vi "Cluster Typedef JSON Staging.vi"(8 "error in (no error)":errorcluster) -> (0 "error out":errorcluster, 1 "Experiment Description 2":T1, 2 "JSON String":string)   [LabVIEW 2016]
uses:
  <userlib>/LevyLab/Lockin-Multichannel/Typedefs/AO-cluster.ctl
  <userlib>/LevyLab/Lockin-Multichannel/Typedefs/AO_Amp-array.ctl
  <userlib>/LevyLab/Lockin-Multichannel/Typedefs/AO_DC-array.ctl
  <userlib>/LevyLab/Lockin-Multichannel/Typedefs/AO_f-array.ctl
  <userlib>/LevyLab/Lockin-Multichannel/Typedefs/AO_phi-array.ctl
  <userlib>/LevyLab/Lockin-Multichannel/Typedefs/Function-array.ctl
  <userlib>/LevyLab/Lockin-Multichannel/Typedefs/Function-enum.ctl
  <userlib>/LevyLab/Krohn Hite 7008/typedefs/KH_control_array.ctl
  <userlib>/LevyLab/Krohn Hite 7008/typedefs/KH_control.ctl
  <userlib>/LevyLab/Krohn Hite 7008/typedefs/Channel-Enum.ctl
  <userlib>/LevyLab/Krohn Hite 7008/typedefs/Gain-Enum.ctl
  <userlib>/LevyLab/Krohn Hite 7008/typedefs/Shunt-Enum.ctl
  <userlib>/LevyLab/Krohn Hite 7008/typedefs/Input Configuration-Enum.ctl
  <userlib>/LevyLab/Lockin-Multichannel/Typedefs/REF-cluster.ctl
  <userlib>/LevyLab/Lockin-Multichannel/Typedefs/REF_f-array.ctl
  <userlib>/LevyLab/Lockin-Multichannel/Typedefs/REF_phi-array.ctl
  <vilib>/addons/_JKI.lib/Serialization/JSON/JKI JSON Serialization.lvlib
  <userlib>/LevyLab/Krohn Hite 7008/KH7008.lvclass
  Control Experiment/Control Experiment.lvclass
panel:
  out "x = y?":T2
  out "from JSON (ms)":u32
  out "to JSON (ms)":u32
  in  "Experiment Description":T1
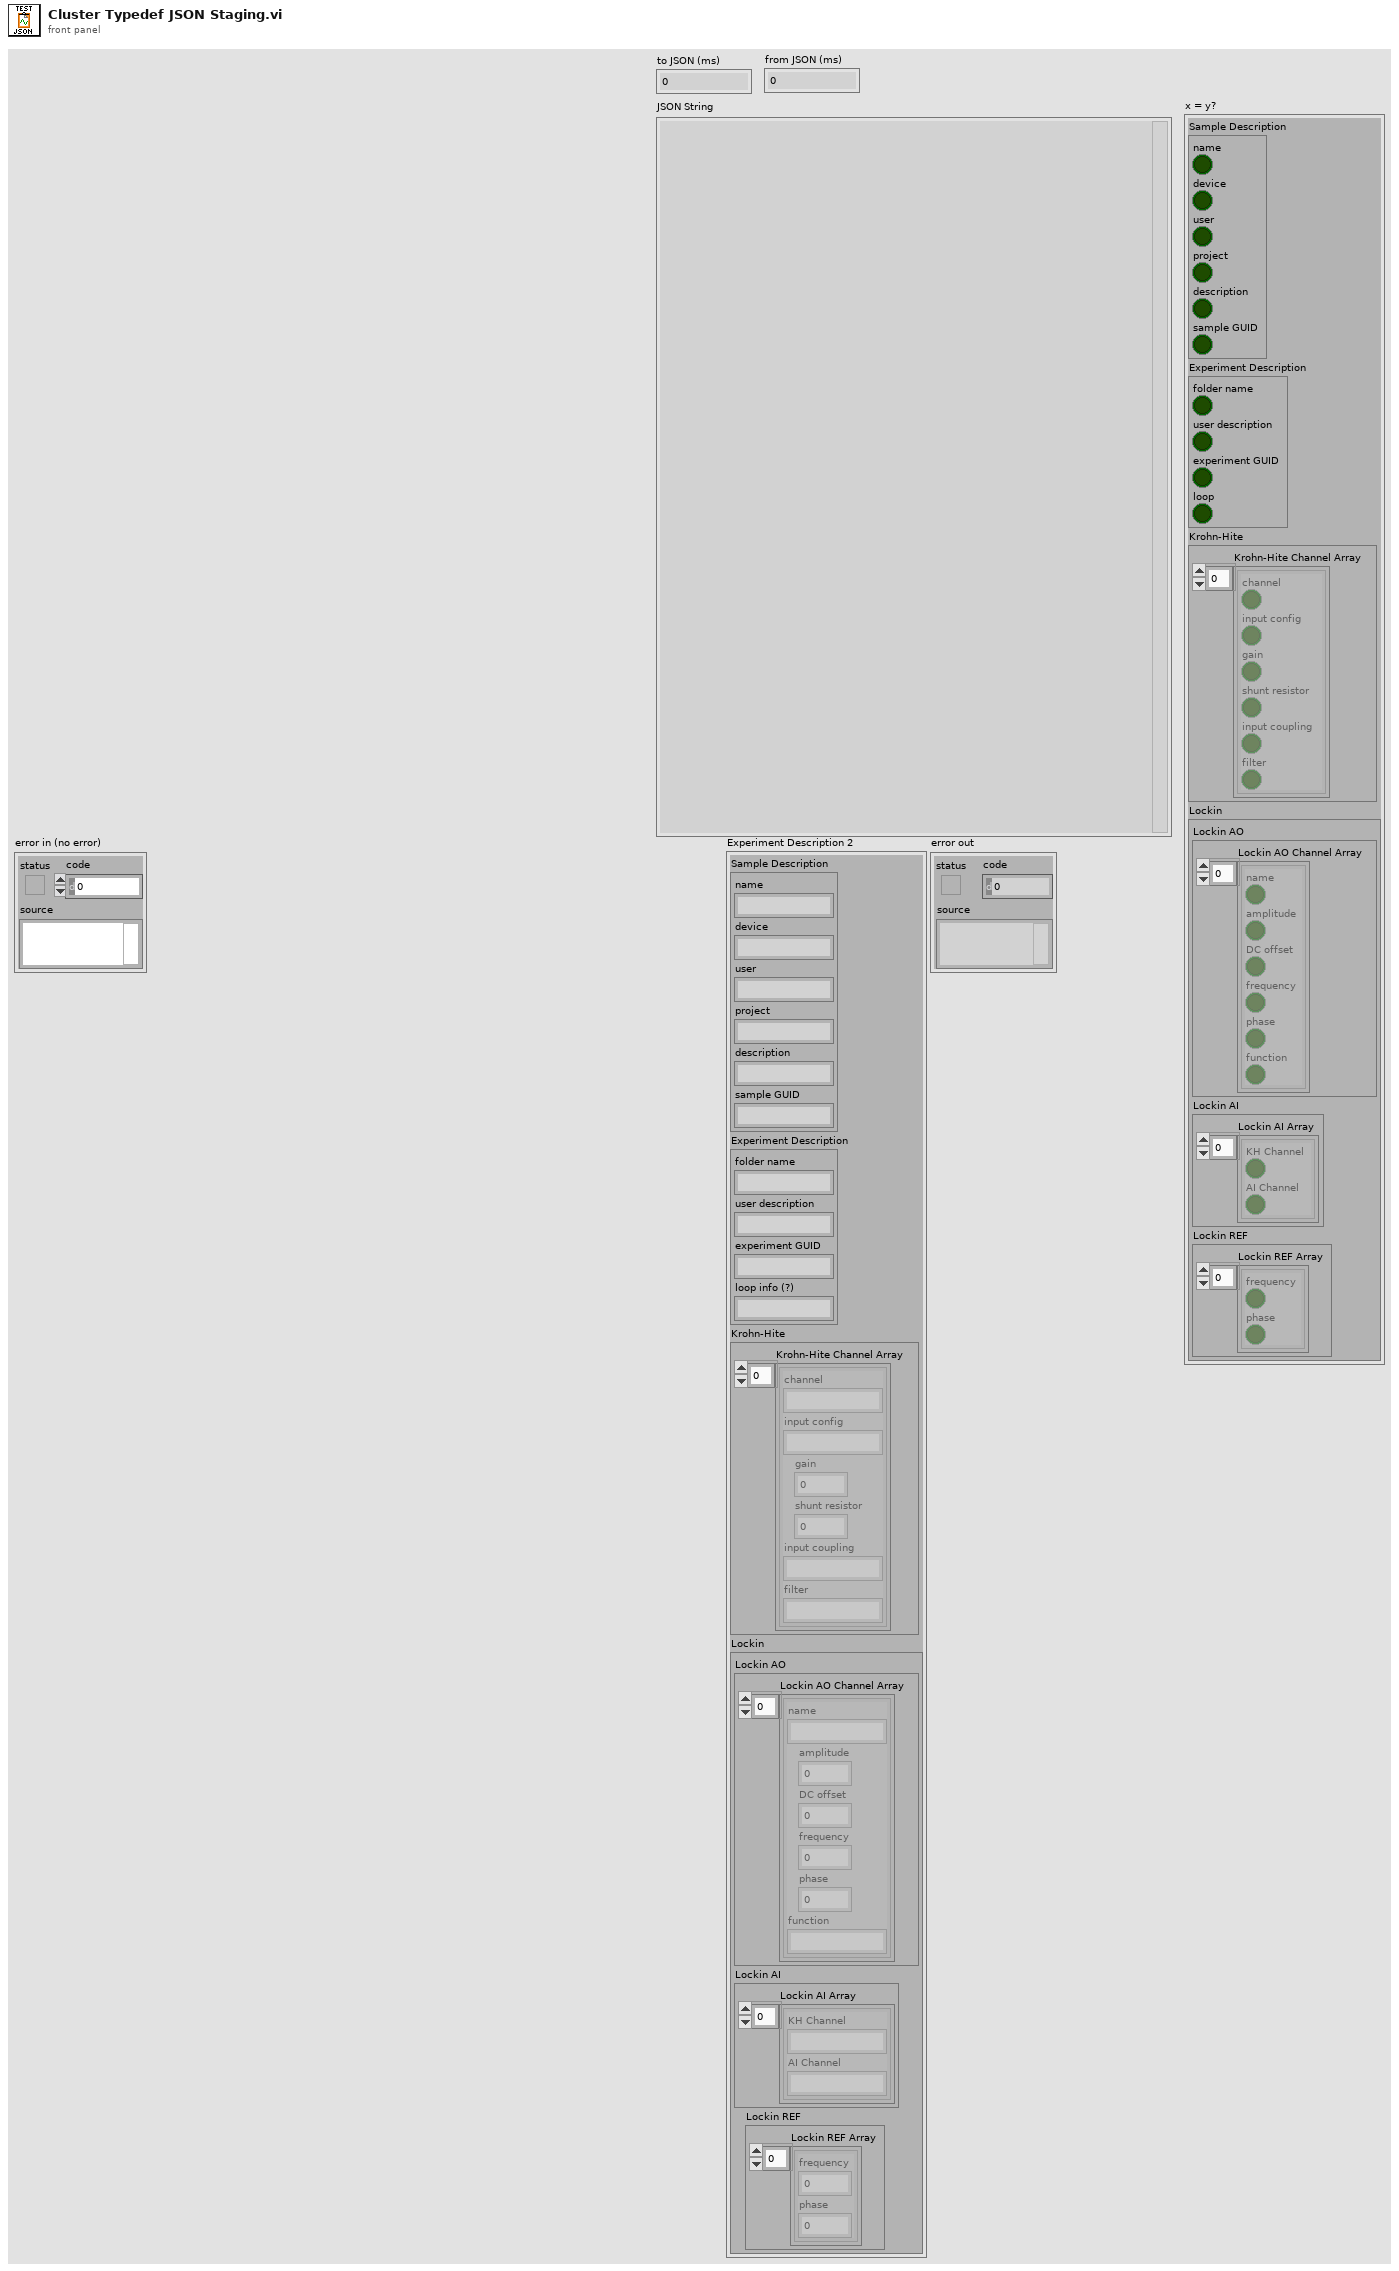
[diagram p1: front panel]
types:
  T1 = cluster{"Sample Description":cluster{"name":string, "device":string, "user":string, "project":string, "description":string, "sample GUID":string}, "Experiment Description":cluster{"folder name":string, "user description":string, "experiment GUID":string, "loop info (?)":string}, "Krohn-Hite":cluster{"Krohn-Hite Channel Array":cluster{"channel":string, "input config":string, "gain":i32, "shunt resistor":i32, "input coupling":string, "filter":string}[]}, "Lockin":cluster{"Lockin AO":cluster{"Lockin AO Channel Array":cluster{"name":string, "amplitude":dbl, "DC offset":dbl, "frequency":dbl, "phase":dbl, "function":string}[]}, "Lockin AI":cluster{"Lockin AI Array":cluster{"KH Channel":string, "AI Channel":string}[]}, "Lockin REF":cluster{"Lockin REF Array":cluster{"frequency":dbl, "phase":dbl}[]}}}
  T2 = cluster{"Sample Description":cluster{"name":bool, "device":bool, "user":bool, "project":bool, "description":bool, "sample GUID":bool}, "Experiment Description":cluster{"folder name":bool, "user description":bool, "experiment GUID":bool, "loop":bool}, "Krohn-Hite":cluster{"Krohn-Hite Channel Array":cluster{"channel":bool, "input config":bool, "gain":bool, "shunt resistor":bool, "input coupling":bool, "filter":bool}[]}, "Lockin":cluster{"Lockin AO":cluster{"Lockin AO Channel Array":cluster{"name":bool, "amplitude":bool, "DC offset":bool, "frequency":bool, "phase":bool, "function":bool}[]}, "Lockin AI":cluster{"Lockin AI Array":cluster{"KH Channel":bool, "AI Channel":bool}[]}, "Lockin REF":cluster{"Lockin REF Array":cluster{"frequency":bool, "phase":bool}[]}}}
  T3 = typedef "REF-cluster.ctl" = cluster{"REF f (Hz)":T4, "REF phi (°)":T5}
  T4 = typedef "REF_f-array.ctl" = dbl[]
  T5 = typedef "REF_phi-array.ctl" = dbl[]
  T6 = typedef "KH7008.lvclass/KH_control_array.ctl" = T7[]
  T7 = typedef "KH7008.lvclass/KH_control.ctl" = cluster{"Channel":T8, "Gain":T9, "Shunt Resistor":T10, "Input Config":T11}
  T8 = typedef "KH7008.lvclass/Channel-Enum.ctl" = enum16{"Channel 1", "Channel 2", "Channel 3", "Channel 4", "Channel 5", "Channel 6", "Channel 7", "Channel 8"}
  T9 = typedef "KH7008.lvclass/Gain-Enum.ctl" = enum16{"1x", "10x", "100x", "1000x"}
  T10 = typedef "KH7008.lvclass/Shunt-Enum.ctl" = enum16{"Open", "50 Ohms", "500 Ohms", "5k Ohms", "50k Ohms"}
  T11 = typedef "KH7008.lvclass/Input Configuration-Enum.ctl" = enum16{"Ground", "SE+ (-gnd)", "SE- (+gnd)", "Differential"}
  T12 = typedef "AO-cluster.ctl" = cluster{"AO amp (V)":T13, "AO DC (V)":T14, "AO f (Hz)":T15, "AO phi (°)":T16, "function":T17, "I+":bool[]}
  T13 = typedef "AO_Amp-array.ctl" = dbl[]
  T14 = typedef "AO_DC-array.ctl" = dbl[]
  T15 = typedef "AO_f-array.ctl" = dbl[]
  T16 = typedef "AO_phi-array.ctl" = dbl[]
  T17 = typedef "Function-array.ctl" = T18[]
  T18 = typedef "Function-enum.ctl" = enum16{"Sine", "Triangle", "Square", "Sawtooth"}
  T19 = cluster{"name":string, "device":string, "user":string, "project":string, "description":string, "sample GUID":string}
  T20 = cluster{"folder name":string, "user description":string, "experiment GUID":string, "loop info (?)":string}
  T21 = cluster{"Krohn-Hite Channel Array":cluster{"channel":string, "input config":string, "gain":i32, "shunt resistor":i32, "input coupling":string, "filter":string}[]}
  T22 = cluster{"Lockin AO":cluster{"Lockin AO Channel Array":cluster{"name":string, "amplitude":dbl, "DC offset":dbl, "frequency":dbl, "phase":dbl, "function":string}[]}, "Lockin AI":cluster{"Lockin AI Array":cluster{"KH Channel":string, "AI Channel":string}[]}, "Lockin REF":cluster{"Lockin REF Array":cluster{"frequency":dbl, "phase":dbl}[]}}
  T23 = cluster{"Lockin AO Channel Array":cluster{"name":string, "amplitude":dbl, "DC offset":dbl, "frequency":dbl, "phase":dbl, "function":string}[]}
  T24 = cluster{"Lockin REF Array":cluster{"frequency":dbl, "phase":dbl}[]}
  T25 = cluster{"Lockin AI Array":cluster{"KH Channel":string, "AI Channel":string}[]}
  T26 = cluster{"channel":string, "input config":string, "gain":i32, "shunt resistor":i32, "input coupling":string, "filter":string}[]
  T27 = cluster{"channel":string, "input config":string, "gain":i32, "shunt resistor":i32, "input coupling":string, "filter":string}
  T28 = cluster{"name":string, "amplitude":dbl, "DC offset":dbl, "frequency":dbl, "phase":dbl, "function":string}[]
  T29 = cluster{"name":string, "amplitude":dbl, "DC offset":dbl, "frequency":dbl, "phase":dbl, "function":string}
  T30 = cluster{"KH Channel":string, "AI Channel":string}[]
  T31 = cluster{"KH Channel":string, "AI Channel":string}
  T32 = cluster{"Sample Description":cluster{"name":bool, "device":bool, "user":bool, "project":bool, "description":bool, "sample GUID":bool}, "Experiment Description":cluster{"folder name":bool, "user description":bool, "experiment GUID":bool, "loop info (?)":bool}, "Krohn-Hite":cluster{"Krohn-Hite Channel Array":cluster{"channel":bool, "input config":bool, "gain":bool, "shunt resistor":bool, "input coupling":bool, "filter":bool}[]}, "Lockin":cluster{"Lockin AO":cluster{"Lockin AO Channel Array":cluster{"name":bool, "amplitude":bool, "DC offset":bool, "frequency":bool, "phase":bool, "function":bool}[]}, "Lockin AI":cluster{"Lockin AI Array":cluster{"KH Channel":bool, "AI Channel":bool}[]}, "Lockin REF":cluster{"Lockin REF Array":cluster{"frequency":bool, "phase":bool}[]}}}
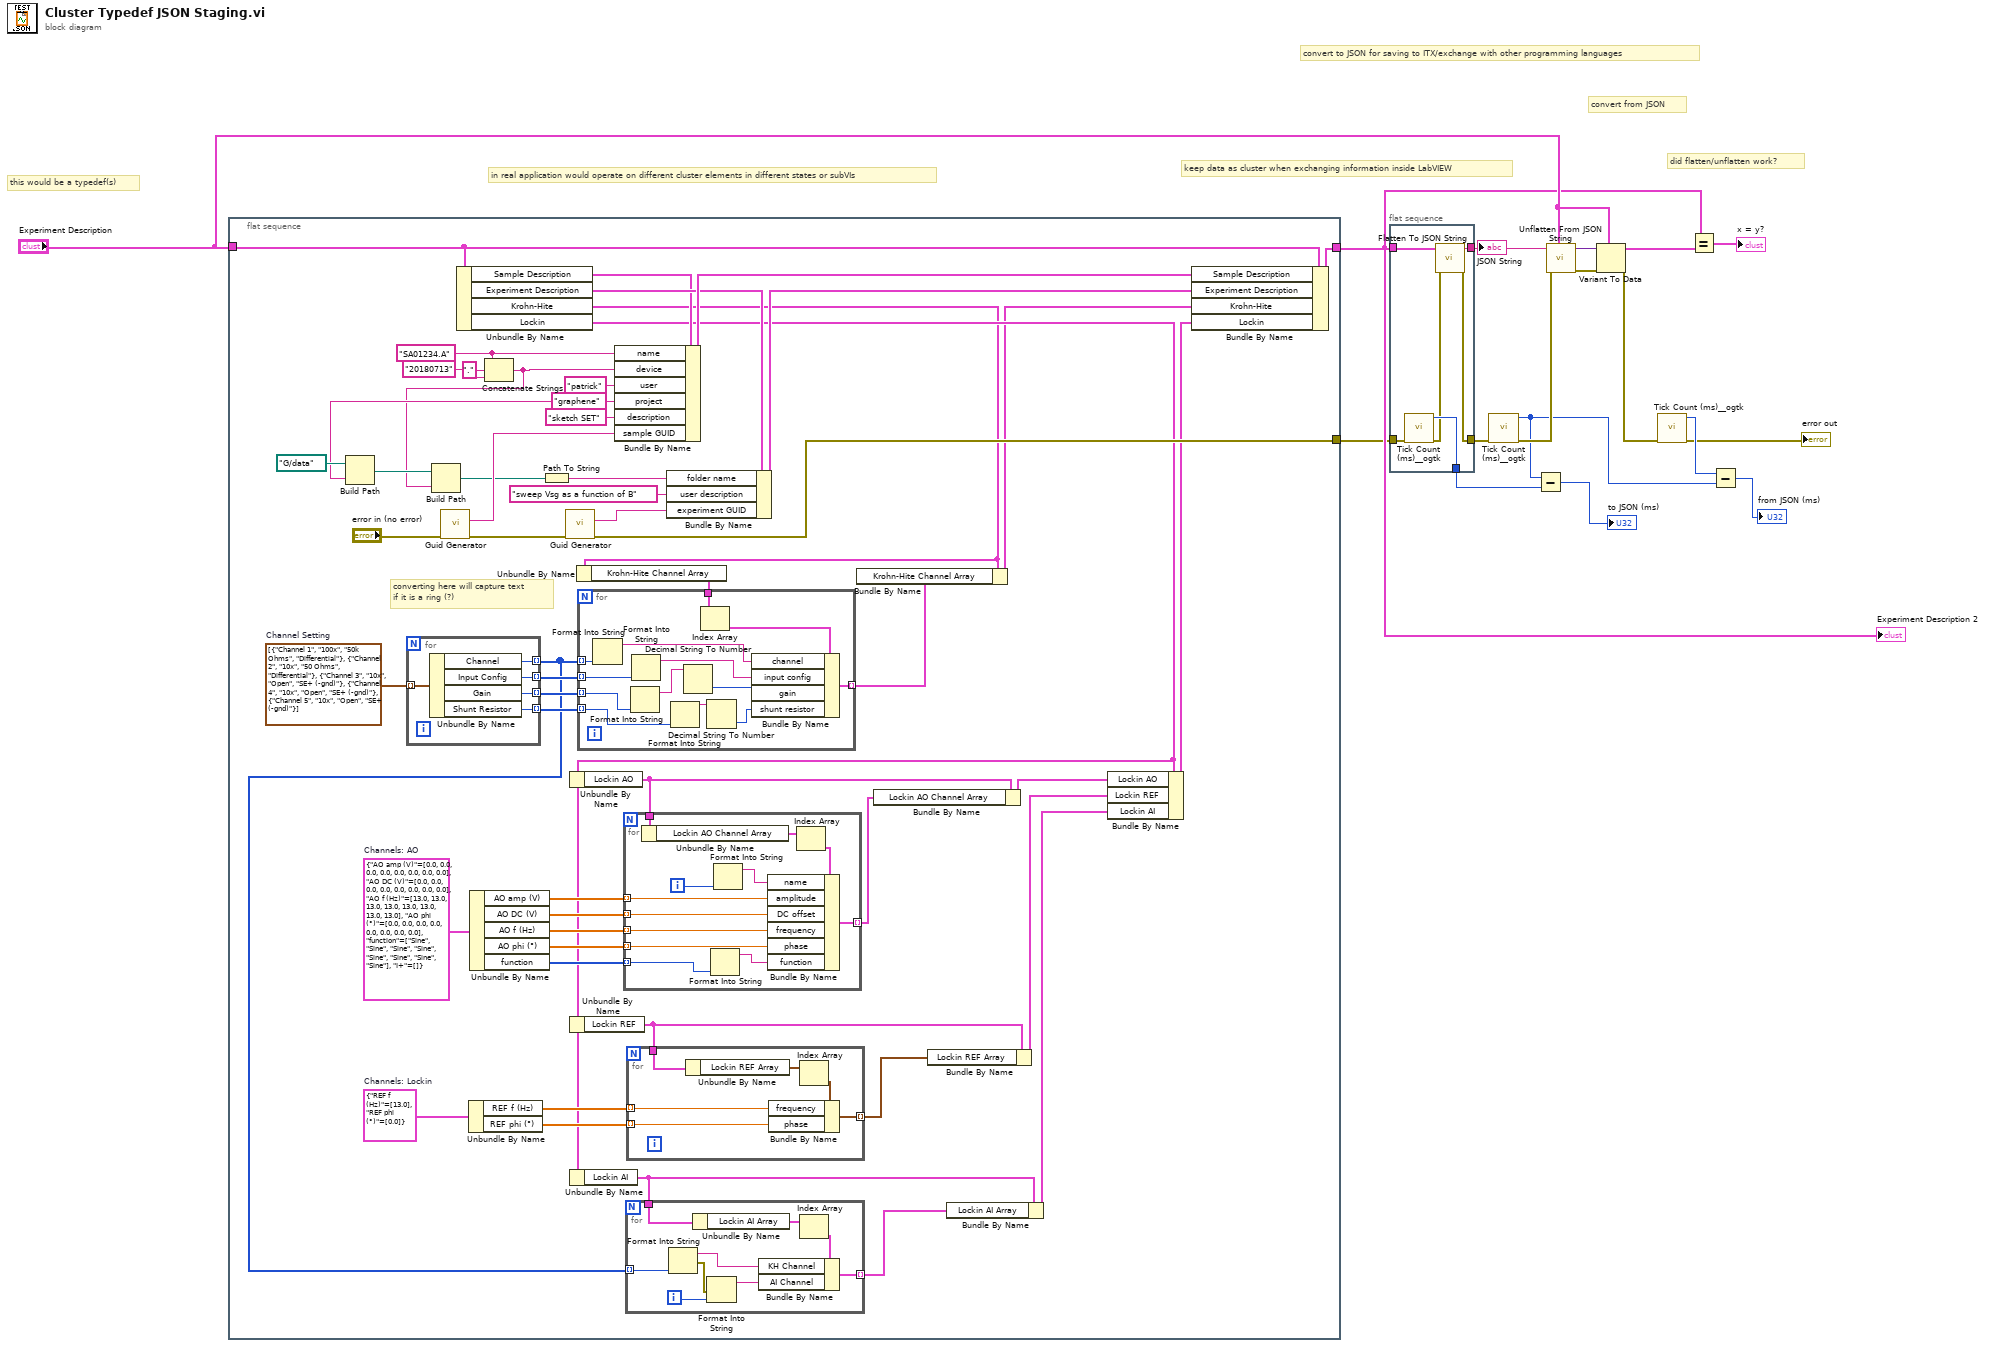
[diagram p0: block diagram]
diagram:
  # "keep data as cluster when exchanging information inside LabVIEW"
  # "did flatten/unflatten work?"
  # "convert from JSON"
  # "convert to JSON for saving to ITX/exchange with other programming languages"
  # "in real application would operate on different cluster elements in different states or subVIs"
  # "this would be a typedef(s)"
  n1 = flat-sequence {
    tunnel: "Experiment Description" -> [w33]
    tunnel: [w32] -> w3
    tunnel: [w24] -> w2
    frame #0 {
      w42 = T3 {"REF f (Hz)"=[13.0], "REF phi (°)"=[0.0]}  # Channels: Lockin
      w48 = "SA01234.A" ("name")
      w35 = "graphene" ("project")
      w68 = T6 [{"Channel"=enum."Channel 1", "Gain"=enum."100x", "Shunt Resistor"=enum."50k Ohms", "Input Config"=enum."Differential"}, {"Channel"=enum."Channel 2", "Gain"=enum."10x", "Shunt Resistor"=enum."50 Ohms", "Input Config"=enum."Differential"}, {"Channel"=enum."Channel 3", "Gain"=enum."10x", "Shunt Resistor"=enum."Open", "Input Config"=enum."SE+ (-gnd)"}, {"Channel"=enum."Channel 4", "Gain"=enum."10x", "Shunt Resistor"=enum."Open", "Input Config"=enum."SE+ (-gnd)"}, {"Channel"=enum."Channel 5", "Gain"=enum."10x", "Shunt Resistor"=enum."Open", "Input Config"=enum."SE+ (-gnd)"}]  # Channel Setting
      w61 = T12 {"AO amp (V)"=[0.0, 0.0, 0.0, 0.0, 0.0, 0.0, 0.0, 0.0], "AO DC (V)"=[0.0, 0.0, 0.0, 0.0, 0.0, 0.0, 0.0, 0.0], "AO f (Hz)"=[13.0, 13.0, 13.0, 13.0, 13.0, 13.0, 13.0, 13.0], "AO phi (°)"=[0.0, 0.0, 0.0, 0.0, 0.0, 0.0, 0.0, 0.0], "function"=[enum."Sine", enum."Sine", enum."Sine", enum."Sine", enum."Sine", enum."Sine", enum."Sine", enum."Sine"], "I+"=[]}  # Channels: AO
      # "converting here will capture text\nif it is a ring (?)"
      n2 = Build Path(base path=path "G:/data", name or relative path=w35) -> (appended path=w45:path)
      n3 = for {
        tunnel: w68 -> [w101] mode=indexing
        tunnel: [w100] -> w28 mode=indexing
        tunnel: [w99] -> w67 mode=indexing
        tunnel: [w98] -> w66 mode=indexing
        tunnel: [w97] -> w65 mode=indexing
        n4 = Unbundle By Name(w101) -> ("Channel"=w100:T8, "Input Config"=w99:T11, "Gain"=w98:T9, "Shunt Resistor"=w97:T10)
      }
      n5 = call "Guid Generator.vi"("error in (no error)"="error in (no error)") -> ("error out"=w23:errorcluster, "GUID"=w46:string)  [unwired: 9 in]
      n6 = Unbundle By Name(w33) -> ("Sample Description"=w29:T19, "Experiment Description"=w30:T20, "Krohn-Hite"=w20:T21, "Lockin"=w21:T22)
      n7 = Unbundle By Name(w42) -> ("REF f (Hz)"=w41:T4, "REF phi (°)"=w40:T5)
      n8 = Unbundle By Name(w61) -> ("AO amp (V)"=w60:T13, "AO DC (V)"=w59:T14, "AO f (Hz)"=w57:T15, "AO phi (°)"=w56:T16, "function"=w55:T17)
      n9 = Concatenate Strings(w48, "." ("string"), "20180713" ("device")) -> (w34:string)
      n10 = Build Path(base path=w45, name or relative path=w34) -> (appended path=w44:path)
      n11 = Path To String(path=w44) -> (string=w43:string)
      n12 = call "Guid Generator.vi"("error in (no error)"=w23) -> ("error out"=w24:errorcluster, "GUID"=w54:string)  [unwired: 9 in]
      n13 = Unbundle By Name(w21) -> ("Lockin AO"=w31:T23)
      n14 = Unbundle By Name(w21) -> ("Lockin REF"=w39:T24)
      n15 = Unbundle By Name(w21) -> ("Lockin AI"=w37:T25)
      n16 = Unbundle By Name(w20) -> ("Krohn-Hite Channel Array"=w63:T26)
      n17 = for {
        tunnel: w63 -> [w111]
        tunnel: [w114] -> w62 mode=indexing
        tunnel: w28 -> [w113] mode=indexing
        tunnel: w67 -> [w112] mode=indexing
        tunnel: w66 -> [w107] mode=indexing
        tunnel: w65 -> [w106] mode=indexing
        n18 = Format Into String(w113) -> (resulting string=w108:string)  [unwired: 3 in, 1 out]
        n19 = Format Into String(w107) -> (resulting string=w104:string)  [unwired: 3 in, 1 out]
        n20 = Format Into String(w112) -> (resulting string=w109:string)  [unwired: 3 in, 1 out]
        n21 = Format Into String(w106) -> (resulting string=w105:string)  [unwired: 3 in, 1 out]
        n22 = Decimal String To Number(string=w104) -> (number=w103:i32)  [unwired: 2 in, 1 out]
        n23 = Index Array(array=w111) -> (element=w110:T27)  [unwired: 1 in]
        n24 = Decimal String To Number(string=w105) -> (number=w102:i32)  [unwired: 2 in, 1 out]
        n25 = Bundle By Name(cluster=w110, "channel"=w108, "input config"=w109, "gain"=w103, "shunt resistor"=w102) -> (w114:T27)
      }
      n26 = Bundle By Name(cluster=w29, "name"=w48, "device"=w34, "user"="patrick", "project"=w35, "description"="sketch SET", "sample GUID"=w46) -> (w64:T19)
      n27 = for {
        tunnel: w31 -> [w92]
        tunnel: [w96] -> w27 mode=indexing
        tunnel: w60 -> [w94] mode=indexing
        tunnel: w59 -> [w93] mode=indexing
        tunnel: w57 -> [w90] mode=indexing
        tunnel: w56 -> [w89] mode=indexing
        tunnel: w55 -> [w88] mode=indexing
        i -> [w95]
        n28 = Unbundle By Name(w92) -> ("Lockin AO Channel Array"=w91:T28)
        n29 = Format Into String(w88) -> (resulting string=w86:string)  [unwired: 3 in, 1 out]
        n30 = Format Into String(w95) -> (resulting string=w87:string)  [unwired: 3 in, 1 out]
        n31 = Index Array(array=w91) -> (element=w85:T29)  [unwired: 1 in]
        n32 = Bundle By Name(cluster=w85, "name"=w87, "amplitude"=w94, "DC offset"=w93, "frequency"=w90, "phase"=w89, "function"=w86) -> (w96:T29)
      }
      n33 = for {
        tunnel: w37 -> [w73]
        tunnel: [w78] -> w25 mode=indexing
        tunnel: w28 -> [w75] mode=indexing
        i -> [w76]
        n34 = Format Into String(w75) -> (resulting string=w74:string, error out=w70:errorcluster)  [unwired: 3 in]
        n35 = Unbundle By Name(w73) -> ("Lockin AI Array"=w77:T30)
        n36 = Format Into String(error in=w70, w76) -> (resulting string=w71:string)  [unwired: 2 in, 1 out]
        n37 = Index Array(array=w77) -> (element=w72:T31)  [unwired: 1 in]
        n38 = Bundle By Name(cluster=w72, "KH Channel"=w74, "AI Channel"=w71) -> (w78:T31)
      }
      n39 = for {
        tunnel: w39 -> [w80]
        tunnel: [w84] -> w26 mode=indexing
        tunnel: w41 -> [w82] mode=indexing
        tunnel: w40 -> [w81] mode=indexing
        n40 = Unbundle By Name(w80) -> ("Lockin REF Array"=w83:cluster{"frequency":dbl, "phase":dbl}[])
        n41 = Index Array(array=w83) -> (element=w79:cluster{"frequency":dbl, "phase":dbl})  [unwired: 1 in]
        n42 = Bundle By Name(cluster=w79, "frequency"=w82, "phase"=w81) -> (w84:cluster{"frequency":dbl, "phase":dbl})
      }
      n43 = Bundle By Name(cluster=w30, "folder name"=w43, "user description"="sweep Vsg as a function of B" ("description"), "experiment GUID"=w54) -> (w69:T20)
      n44 = Bundle By Name(cluster=w20, "Krohn-Hite Channel Array"=w62) -> (w19:T21)
      n45 = Bundle By Name(cluster=w31, "Lockin AO Channel Array"=w27) -> (w58:T23)
      n46 = Bundle By Name(cluster=w39, "Lockin REF Array"=w26) -> (w38:T24)
      n47 = Bundle By Name(cluster=w37, "Lockin AI Array"=w25) -> (w36:T25)
      n48 = Bundle By Name(cluster=w21, "Lockin AO"=w58, "Lockin REF"=w38, "Lockin AI"=w36) -> (w18:T22)
      n49 = Bundle By Name(cluster=w33, "Sample Description"=w64, "Experiment Description"=w69, "Krohn-Hite"=w19, "Lockin"=w18) -> (w32:T1)
    }
  }
  n50 = flat-sequence {
    tunnel: [w120] -> w17
    tunnel: [w119] -> w14
    tunnel: w3 -> [w118]
    tunnel: [w117] -> w8
    tunnel: w2 -> [w115]
    frame #0 {
      n51 = call <userlib>:"Tick Count (ms)__ogtk.vi"("error in (no error)"=w115) -> ("error out"=w116:errorcluster, "millisecond timer value"=w117:u32)  [unwired: 9 in]
      n52 = call <vilib>:"Flatten To JSON String.vi"("error in (no error)"=w116, "Variant"=w118) -> ("error out"=w119:errorcluster, "JSON String"=w120:string)  [unwired: 8 in]
    }
  }
  n53 = call <userlib>:"Tick Count (ms)__ogtk.vi"("error in (no error)"=w14) -> ("error out"=w13:errorcluster, "millisecond timer value"=w6:u32)  [unwired: 9 in]
  n54 = Subtract(x=w6, y=w8) -> (x-y=→"to JSON (ms)":u32)
  n55 = call <vilib>:"Unflatten From JSON String.vi"("Type and Defaults"="Experiment Description", "error in (no error)"=w13, "JSON String"=w17) -> ("error out"=w16:errorcluster, "Variant"=w15:variant)  [unwired: 7 in]
  n56 = Variant To Data(error in=w16, type="Experiment Description", Variant=w15) -> (data=w9:T1, error out=w12:errorcluster)
  n57 = call <userlib>:"Tick Count (ms)__ogtk.vi"("error in (no error)"=w12) -> ("error out"=→"error out":errorcluster, "millisecond timer value"=w7:u32)  [unwired: 9 in]
  n58 = Equal?(x=w3, y=w9) -> (x = y?=→"x = y?":T32)
  n59 = Subtract(x=w7, y=w6) -> (x-y=→"from JSON (ms)":u32)
  "JSON String" <- w17
  "Experiment Description 2" <- w3
